vi "Test Static Test Method 1.vi"(8 "error in (no error)":errorcluster, 11 "Test Case In":refnum<class "My Test Case.lvclass">) -> (0 "error out":errorcluster, 3 "Test Case Out":refnum<class "My Test Case.lvclass">)   [LabVIEW 2020, in "My Test Case.lvclass"]
uses:
  My Test Case.lvclass
  My Test Case.lvclass/My Test Case.ctl
  01074fa8-ee8a-411d-bc8b-fc92c4f90959.vi
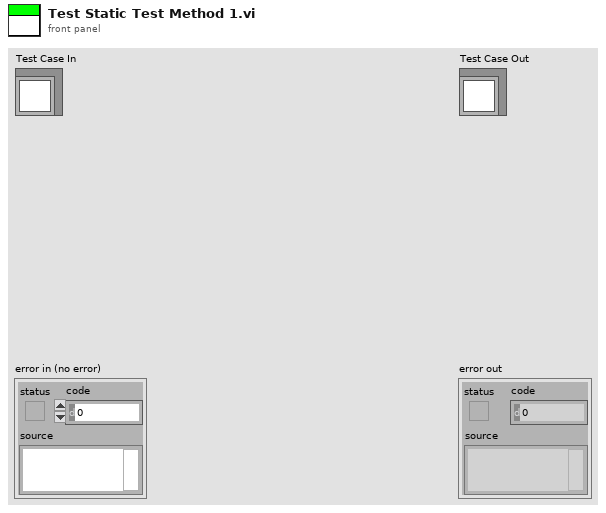
[diagram p1: front panel]
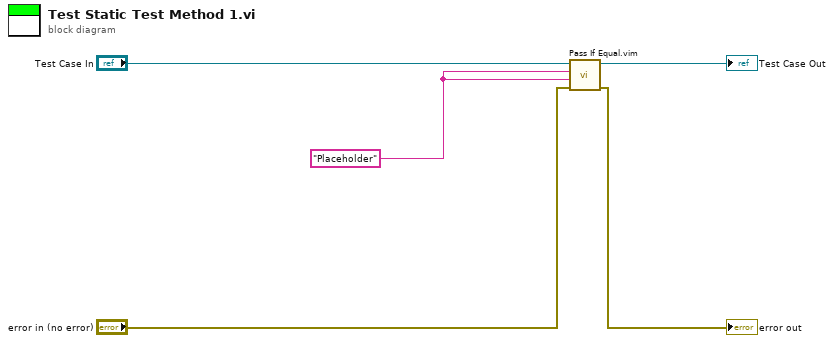
[diagram p0: block diagram]
diagram:
  w1 = "Placeholder"
  n1 = call "Pass If Equal.vim"("error in (no error)"="error in (no error)", "Actual"=w1, "Expected"=w1, "LUnit Test Case In"="Test Case In") -> ("error out"=→"error out":errorcluster, "LUnit Test Case Out"=→"Test Case Out":refnum<class "My Test Case.lvclass">)  [unwired: 6 in]
